vi "Part 2.vi"(11 "Input":string) -> (3 "Output":i64)   [LabVIEW 2021]
uses:
  <userlib>/_OpenG.lib/string/string.llb/Convert EOLs (String)__ogtk.vi
panel:
  out "Nodes":cluster{i32, i32}[](array[cluster])
  out "Start":cluster{"Row":i32, "Col":i32}
  out "End":cluster{"Row":i32, "Col":i32}
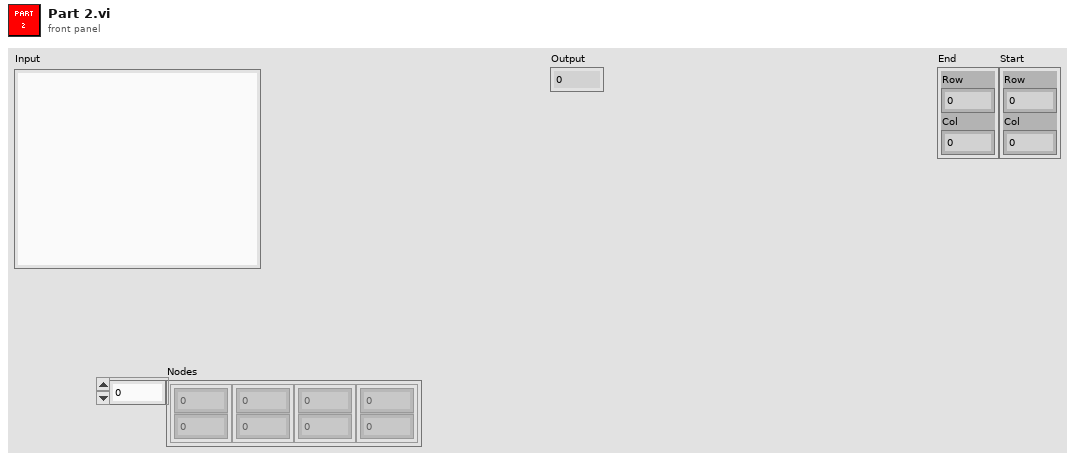
[diagram p1: front panel]
types:
  T1 = map{cluster{i32, i32}, cluster{"Node":cluster{i32, i32}, "Distance":i64}[]}
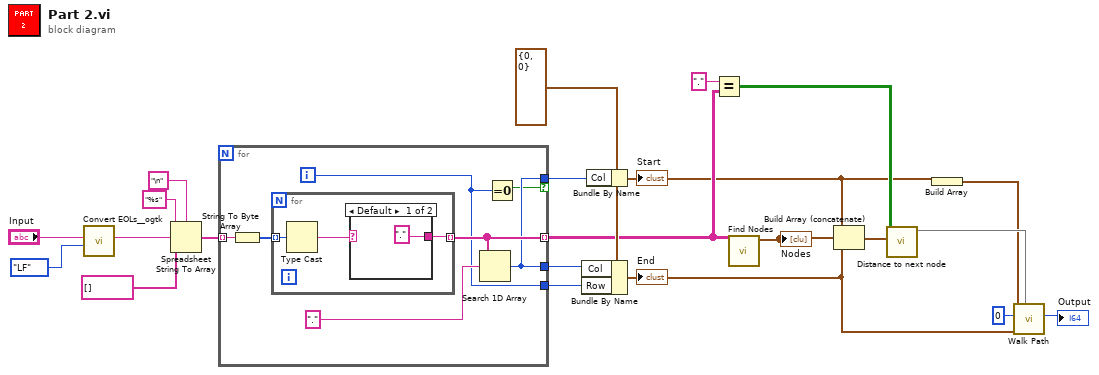
[diagram p0: block diagram]
diagram:
  w14 = cluster{"Row":i32, "Col":i32} {"Row"=0, "Col"=0}
  n1 = call-poly <userlib>:"Convert EOLs__ogtk.vi"("Convert to:"=enum16{"CR", "LF", "CRLF"}."LF", "String in"="Input") -> ("String out"=w18:string)  [unwired: 9 in]
  n2 = Spreadsheet String To Array(delimiter (Tab)="\n", format string="%s", spreadsheet string=w18, array type (2D Dbl)=string[] []) -> (array=w16:string[])
  n3 = for {
    tunnel: w16 -> [w29] mode=indexing
    tunnel: [w27] -> w10 mode=indexing
    tunnel: [w25] -> w13
    tunnel: [w25] -> w15 if=w24
    tunnel: [w23] -> w12
    i -> [w23]
    n4 = String To Byte Array(string=w29) -> (unsigned byte array=w28:u8[])
    n5 = for {
      tunnel: w28 -> [w32] mode=indexing
      tunnel: [w30] -> w27 mode=indexing
      n6 = Type Cast(x=w32) -> (*(type *) &x=w31:string)  [unwired: 1 in]
      n7 = case shown="Default" w31 {
        selector: w31 -> [_ w34]
        tunnel: ["." w34] -> w30
        frame Default {
        }
        frame "#" {
        }
      }
    }
    n8 = Search 1D Array(1D array=w27, element=".") -> (index of element=w25:i32)  [unwired: 1 in]
    n9 = Equal To 0?(x=w23) -> (x = 0?=w24:bool)
  }
  n10 = Bundle By Name(cluster=w14, "Col"=w13, "Row"=w12) -> (w6:cluster{"Row":i32, "Col":i32})
  "End" <- w6
  n11 = Bundle By Name(cluster=w14, "Col"=w15) -> (w3:cluster{"Row":i32, "Col":i32})
  "Start" <- w3
  n12 = Equal?(x=".", y=w10) -> (x = y?=w8:bool[][])
  n13 = call "Find Nodes.vi"("Array in"=w10) -> ("Array out"=w9:cluster{i32, i32}[])  [unwired: 10 in]
  "Nodes" <- w9
  n14 = Build Array (concatenate)(w3, w9, w6) -> (w7:cluster{"Row":i32, "Col":i32}[])
  n15 = call "Distance to next node.vi"("Nodes"=w7, "Grid"=w8) -> ("Next Node Map"=w5:T1)  [unwired: 9 in]
  n16 = Build Array(w3) -> (w2:cluster{"Row":i32, "Col":i32}[])
  n17 = call "Walk Path.vi"("Next Node Map"=w5, "End"=w6, "Distance In"=i64 0, "Path In"=w2) -> ("Distance Out"=→"Output":i64)  [unwired: 7 in]
